vi "Create Evaluation String.vi"(8 "error in (no error)":errorcluster, 10 "Evaluation String":string, 11 "Str Equal in":refnum<class "Str Equal.lvclass">) -> (0 "error out":errorcluster, 3 "Str Equal out":refnum<class "Str Equal.lvclass">)   [LabVIEW 2018, in "Str Equal.lvclass"]
uses:
  Str Equal.lvclass
  C:/Users/UKHornP/Documents/Work/Projects/Assert API/Plugins/Utility/Test Classes/Test.lvclass
  String.lvclass
  Test.lvclass
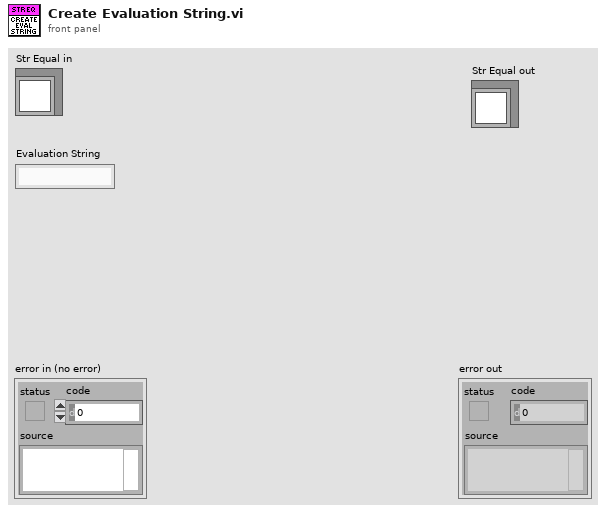
[diagram p1: front panel]
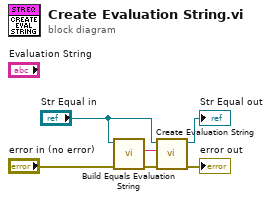
[diagram p0: block diagram]
diagram:
  n1 = call "Build Equals Evaluation String.vi"("error in (no error)"="error in (no error)", "Test in"="Str Equal in") -> ("error out"=w1:errorcluster, "Equals Evaluation String"=w2:string)  [unwired: 8 in]
  n2 = call-parent "Create Evaluation String.vi"("error in (no error)"=w1, "Evaluation String"=w2, "String in"="Str Equal in") -> ("error out"=→"error out":errorcluster, "String out"=→"Str Equal out":refnum<class "Str Equal.lvclass">)  [unwired: 7 in]
